vi "solar_voy EnQ (Error).vi"(7 "Setup":T1, 8 "error in (no error)":errorcluster, 11 "Voyager Refnum in":T2) -> (0 "error out":errorcluster, 3 "Voyager Refnum out":T2)   [LabVIEW 2018]
doc: "This enqueues the error to the default Target."
uses:
  solar_voy_ctl Port Setup.ctl
  solar_voy_ctl Voyager Refnum.ctl
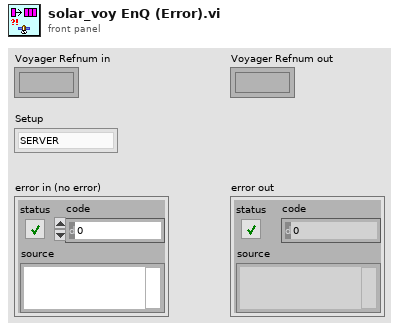
[diagram p1: front panel]
types:
  T1 = typedef "solar_voy_ctl Port Setup.ctl" = enum8{"SERVER", "CLIENT", "SERVER_CMD", "SERVER_TLM"}
  T2 = typedef "solar_voy_ctl Voyager Refnum.ctl" = refnum<k1>
  T3 = typedef "solar_voy_ctl Voyager.ctl" = cluster{"PACKETS":T4[], "COSMOS_Root":path, "CMD_HDR":T9, "TLM_HDR":T9, "TCPs":T10[], "VoyagerIDOffset":cluster{"VoyagerIDOffset":u16[], "Target Names":string[]}}
  T4 = typedef "solar_voy_def_ctl PACKET.ctl" = cluster{"PACKET_ID":T5, "ENDIAN":enum8{"BIG", "LITTLE"}, "DESC":string, "HZRD":bool, "ITEMS":T6[], "NoExport":bool, "last_time":timestamp, "last_count":u32, "last_data":string}
  T5 = typedef "solar_voy_def_ctl PACKET_ID.ctl" = cluster{"ID":u16, "CMD":enum8{"CMD", "TLM"}, "TARGET":string, "PACKET":string}
  T6 = typedef "solar_voy_def_ctl ITEM.ctl" = cluster{"NAME":string, "OFFSET":i32, "SIZE":i32, "TYPE":T7, "EACH_SIZE":i32, "LVTYPE":T8, "MIN":dbl, "MAX":dbl, "DEFAULT":string, "DESC":string, "ID":bool, "MODIFIERS":variant, "last_value":variant}
  T7 = typedef "solar_voy_def_ctl ITEM TYPE.ctl" = enum8{"BLOCK", "INT", "UINT", "FLOAT", "STRING"}
  T8 = typedef "solar_type Item Type.ctl" = enum16{"NULL", "UNKNOWN", "CLUSTER", "I8", "I16", "I32", "I64", "U8", "U16", "U32", "U64", "U8_ENUM", "U16_ENUM", "U32_ENUM", "SGL", "DBL", "BOOLEAN", "STRING", "PATH", "VISA", "TAG", "TIME", "I8_1D", "I16_1D", "I32_1D", "I64_1D", "U8_1D", "U16_1D", "U32_1D", "U64_1D", "U8_ENUM_1D", "U16_ENUM_1D", "U32_ENUM_1D", "SGL_1D", "DBL_1D", "BOOLEAN_1D", "STRING_1D", "PATH_1D", "VISA_1D", "TAG_1D", "TIME_1D", "I8_2D", "I16_2D", "I32_2D", "I64_2D", "U8_2D", "U16_2D", "U32_2D", "U64_2D", "U8_ENUM_2D", "U16_ENUM_2D", "U32_ENUM_2D", "SGL_2D", "DBL_2D", "BOOLEAN_2D", "STRING_2D", "PATH_2D", "VISA_2D", "TAG_2D", "TIME_2D"}
  T9 = typedef "solar_voy_def_ctl HDR.ctl" = cluster{"ITEMS":T6[], "LENGTH_NAME":string, "LENGTH_VALUE_OFFSET":i32, "ID_NAME":string, "ENDIAN":enum8{"BIG", "LITTLE"}, "GUID_NAME":string, "DEFAULT_TARGET":string, "DEFAULT_PACKET":string, "DEFAULT_ERROR":string}
  T10 = typedef "solar_voy_ctl TCP.ctl" = cluster{"Connected":bool, "Port":u16, "Listener":refnum<k5>, "ServerIP":string, "TCP":refnum<k5>, "Setup":T1, "VIRefnum":refnum<vi>, "TARGETS_CMD":string[], "TARGETS_TLM":string[]}
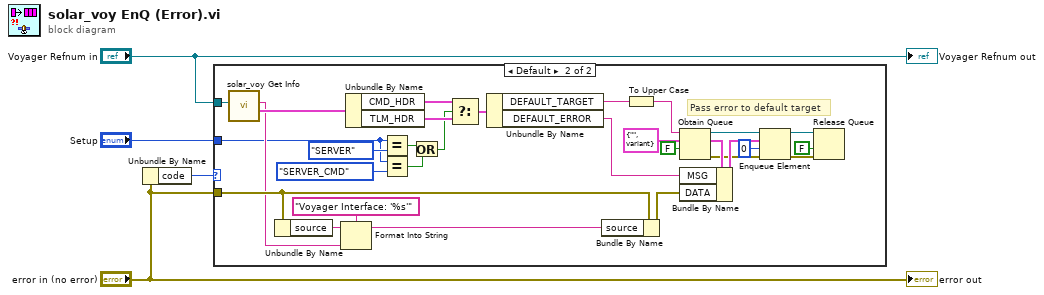
[diagram p0: block diagram]
diagram:
  n1 = Unbundle By Name("error in (no error)") -> ("code"=w2:i32)
  n2 = case shown="Default" w2 {
    tunnel: "Voyager Refnum in" -> [_ w33]
    tunnel: "error in (no error)" -> [_ w22]
    tunnel: "Setup" -> [_ w5]
    frame 0 {
    }
    frame Default {
      w30 = cluster{"MSG":string, "DATA":variant} {"MSG"="", "DATA"=variant} ("MSG")
      # "Pass error to default target"
      n3 = call "solar_voy Get Info.vi"("Voyager Refnum"=w33) -> ("Voyager"=w23:T3, "Interface Name"=w18:string)  [unwired: 8 in, 1 out]
      n4 = Unbundle By Name(w22) -> ("source"=w17:string)
      n5 = Format Into String(format string="Voyager Interface: '%s'", initial string=w17, w18) -> (resulting string=w20:string)  [unwired: 1 in, 1 out]
      n6 = Unbundle By Name(w23) -> ("CMD_HDR"=w16:T9, "TLM_HDR"=w15:T9)
      n7 = Equal?(x=w5, y=solar_voy_ctl_Port_Setup."SERVER") -> (x = y?=w10:bool)
      n8 = Equal?(x=w5, y=solar_voy_ctl_Port_Setup."SERVER_CMD") -> (x = y?=w7:bool)
      n9 = Or(x=w10, y=w7) -> (x .or. y?=w6:bool)
      n10 = Select(t=w16, s=w6, f=w15) -> (s? t:f=w14:T9)
      n11 = Unbundle By Name(w14) -> ("DEFAULT_TARGET"=w12:string, "DEFAULT_ERROR"=w13:string)
      n12 = Bundle By Name(cluster=w22, "source"=w20) -> (w21:errorcluster)
      n13 = To Upper Case(1:w12) -> (0:w11:string)
      n14 = Obtain Queue(name (unnamed)=w11, element data type=w30, create if not found? (T)=FALSE) -> (queue out=w24:refnum<queue>, error out=w29:errorcluster)  [unwired: 2 in, 1 out]
      n15 = Bundle By Name(cluster=w30, "MSG"=w13, "DATA"=w21) -> (w31:cluster{"MSG":string, "DATA":variant})
      n16 = Enqueue Element(queue=w24, element=w31, timeout in ms (-1)=0, error in (no error)=w29) -> (queue out=w27:refnum<queue>, error out=w28:errorcluster)  [unwired: 1 out]
      n17 = Release Queue(queue=w27, force destroy? (F)=FALSE, error in (no error)=w28) -> ()  [unwired: 3 out]
    }
  }
  "Voyager Refnum out" <- "Voyager Refnum in"
  "error out" <- "error in (no error)"
